vi "CameraKill.vi"(8 "error in (no error)":errorcluster, 11 "CameraBase in":refnum<class "CameraBase.lvclass">) -> (0 "error out":errorcluster, 3 "CameraBase out":refnum<class "CameraBase.lvclass">)   [LabVIEW 2012, in "CameraBase.lvclass"]
uses:
  <userlib>/BIAS2/classes/CameraBase/CameraBase.lvclass
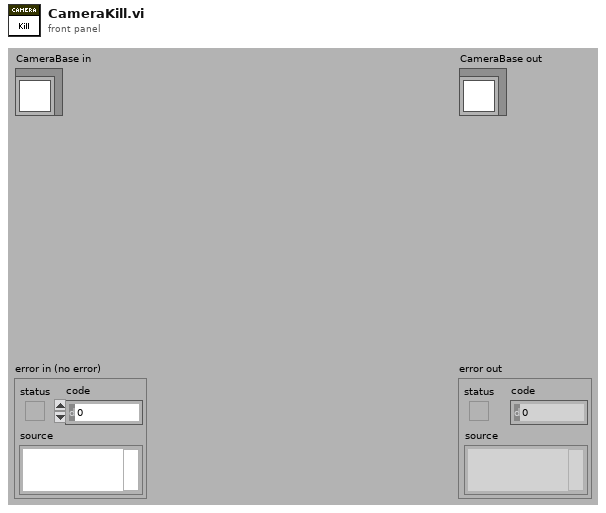
[diagram p1: front panel]
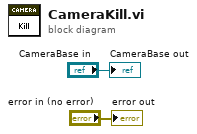
[diagram p0: block diagram]
diagram:
  "error out" <- "error in (no error)"
  "CameraBase out" <- "CameraBase in"
